vi "AIT 664 - Read 664 Device XML.vi"(0 "Refnum in":refnum<k20>, 11 "error in (no error)":errorcluster) -> (4 "Refnum out":refnum<k20>, 6 "664 Device":T1, 15 "error out":errorcluster)   [LabVIEW 2013, in "AIT 664 Custom Device.lvlib"]
doc: "Read <a664Device> information from XML file"
uses:
  AIT 664 Custom Device.lvlib
  Controls/664 - XML Device Description.ctl
  Controls/664 - XML End System Description.ctl
  Controls/664 - XML Output VL.ctl
  Controls/664 - XML Tx Message Port.ctl
  Controls/664 - Sampling Type.ctl
  Controls/664 -Param.ctl
  Controls/664 - XML Input VL.ctl
  Controls/664 - XML Rx Message Port.ctl
  <vilib>/xml/Close Reference(NNMap).vi
  <resource>/objmgr/DOMUserDefRef.rc
  <vilib>/xml/NI_XML.lvlib
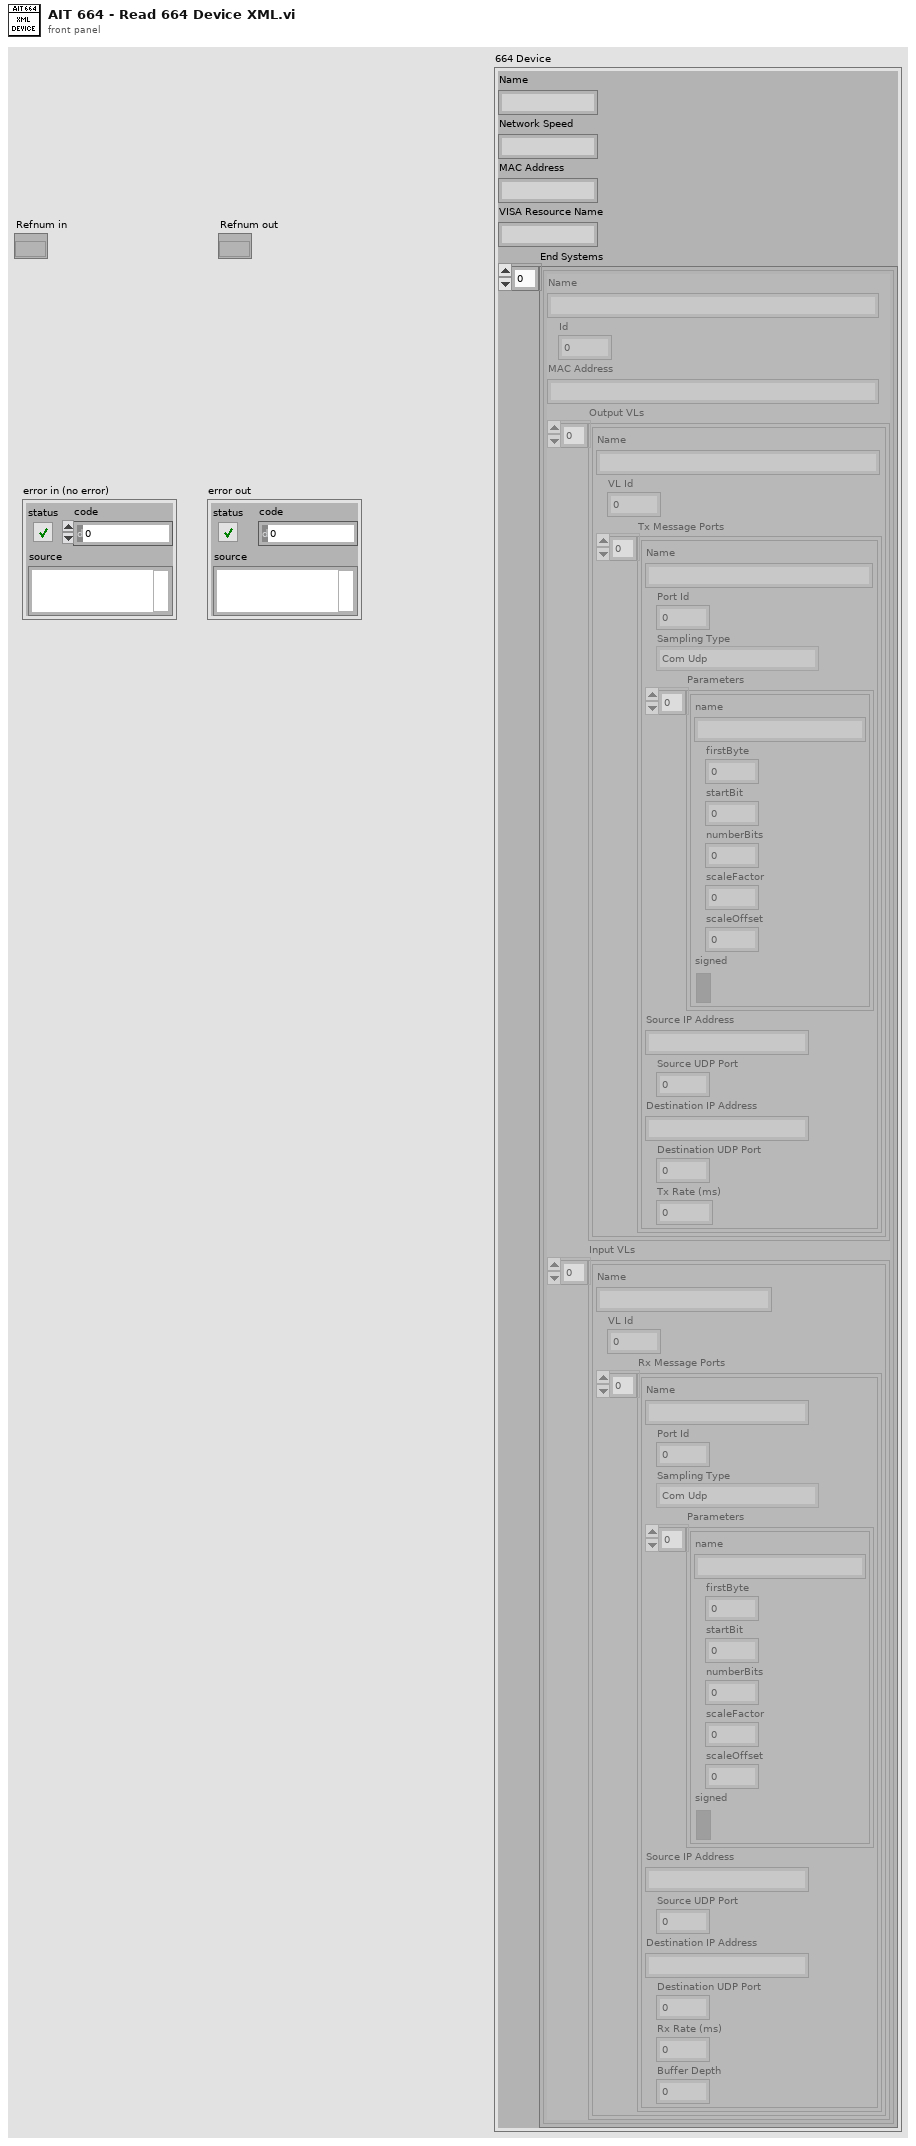
[diagram p1: front panel]
types:
  T1 = typedef "AIT 664 Custom Device.lvlib/664 - XML Device Description.ctl" = cluster{"Name":string, "Network Speed":string, "MAC Address":string, "VISA Resource Name":string, "End Systems":T2[]}
  T2 = typedef "AIT 664 Custom Device.lvlib/664 - XML End System Description.ctl" = cluster{"Name":string, "Id":u32, "MAC Address":string, "Output VLs":T3[], "Input VLs":T7[]}
  T3 = typedef "AIT 664 Custom Device.lvlib/664 - XML Output VL.ctl" = cluster{"Name":string, "VL Id":u32, "Tx Message Ports":T4[]}
  T4 = typedef "AIT 664 Custom Device.lvlib/664 - XML Tx Message Port.ctl" = cluster{"Name":string, "Port Id":u32, "Sampling Type":T5, "Parameters":T6[], "Source IP Address":string, "Source UDP Port":u32, "Destination IP Address":string, "Destination UDP Port":u32, "Tx Rate (ms)":u32}
  T5 = typedef "AIT 664 Custom Device.lvlib/664 - Sampling Type.ctl" = enum16{"Com Udp", "Com Udp Queuing", "Sap Udp", "Sap Ip", "Sap Mac", "Unknown"}
  T6 = typedef "AIT 664 Custom Device.lvlib/664 -Param.ctl" = cluster{"name":string, "firstByte":i32, "startBit":i32, "numberBits":i32, "scaleFactor":dbl, "scaleOffset":dbl, "signed":bool}
  T7 = typedef "AIT 664 Custom Device.lvlib/664 - XML Input VL.ctl" = cluster{"Name":string, "VL Id":u32, "Rx Message Ports":T8[]}
  T8 = typedef "AIT 664 Custom Device.lvlib/664 - XML Rx Message Port.ctl" = cluster{"Name":string, "Port Id":u32, "Sampling Type":T5, "Parameters":T6[], "Source IP Address":string, "Source UDP Port":u32, "Destination IP Address":string, "Destination UDP Port":u32, "Rx Rate (ms)":u32, "Buffer Depth":u32}
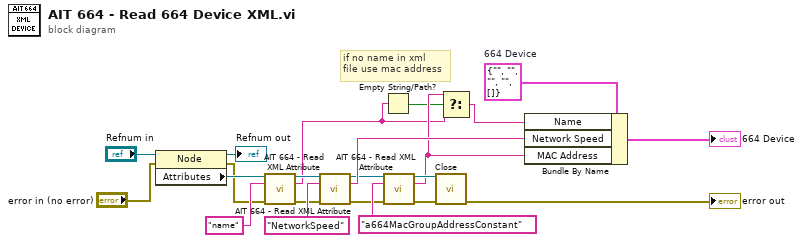
[diagram p0: block diagram]
diagram:
  w20 = T1 {"Name"="", "Network Speed"="", "MAC Address"="", "VISA Resource Name"="", "End Systems"=[]}  # 664 Device
  # "if no name in xml\nfile use mac address"
  n1 = property class="Node"(reference="Refnum in", error in="error in (no error)") -> (reference out=→"Refnum out":refnum<k20>, error out=w7:errorcluster, "Attributes"=w8:refnum<k20>)
  n2 = call "AIT 664 - Read XML Attribute.vi"("Attributes In"=w8, "Attribute Name"="name" ("Name"), "error in (no error)"=w7) -> ("Attributes Out"=w10:refnum<k20>, "Attribute Text"=w2:string, "error out"=w11:errorcluster)  [unwired: 10 in]
  n3 = call "AIT 664 - Read XML Attribute.vi"("Attributes In"=w10, "Attribute Name"="NetworkSpeed" ("Name"), "error in (no error)"=w11) -> ("Attributes Out"=w14:refnum<k20>, "Attribute Text"=w21:string, "error out"=w13:errorcluster)  [unwired: 10 in]
  n4 = Empty String/Path?(string/path=w2) -> (empty?=w1:bool)
  n5 = call "AIT 664 - Read XML Attribute.vi"("Attributes In"=w14, "Attribute Name"="a664MacGroupAddressConstant" ("Name"), "error in (no error)"=w13) -> ("Attributes Out"=w16:refnum<k20>, "Attribute Text"=w4:string, "error out"=w15:errorcluster)  [unwired: 10 in]
  n6 = call-poly <vilib>:"Close.vi"("error in (no error)"=w15, "named node map"=w16) -> ("error out"=→"error out":errorcluster)  [unwired: 7 in]
  n7 = Select(t=w4, s=w1, f=w2) -> (s? t:f=w3:string)
  n8 = Bundle By Name(cluster=w20, "Name"=w3, "Network Speed"=w21, "MAC Address"=w4) -> (→"664 Device":T1)
